vi "MEMR-Export Gain Spectra.vi"(0 "path":path=path "D:/Data/MEMR/Ken/SFMH41-MEMR-1.txt", 7 "processed":T1) -> (15 "error out":errorcluster)   [LabVIEW 2020]
uses:
  Analysis VIs/MEMR-Processed Data.ctl
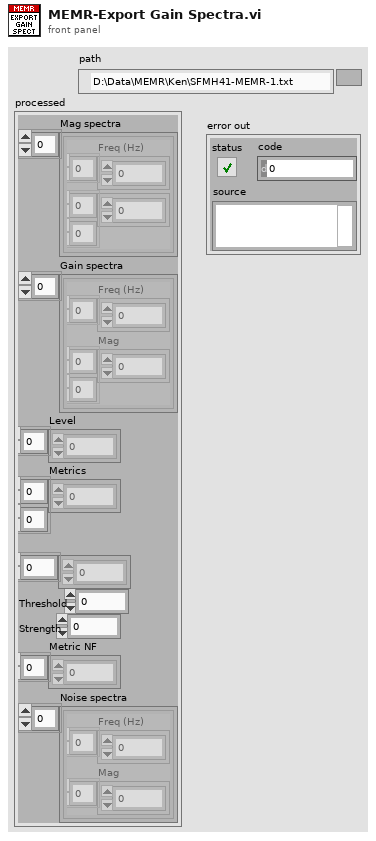
[diagram p1: front panel]
types:
  T1 = typedef "MEMR-Processed Data.ctl" = cluster{"Mag spectra":cluster{"Freq (Hz)":dbl[], dbl[][]}[], "Gain spectra":cluster{"Freq (Hz)":dbl[], "Mag":dbl[][]}[], "Level":dbl[], "Metrics":dbl[][], "Fpeak":dbl[], "Threshold":dbl, "Strength":dbl, "Metric NF":dbl[], "Noise spectra":cluster{"Freq (Hz)":dbl[], "Mag":dbl[]}[]}
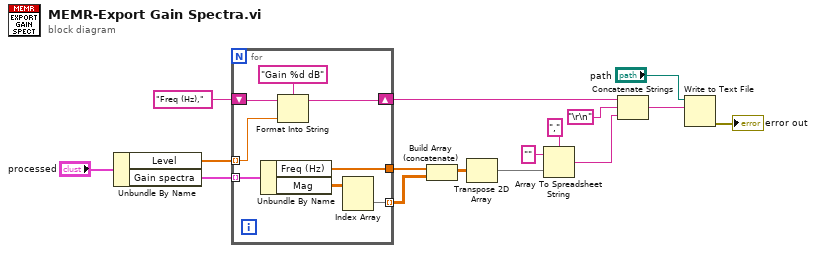
[diagram p0: block diagram]
diagram:
  n1 = Unbundle By Name("processed") -> ("Level"=w14:dbl[], "Gain spectra"=w15:cluster{"Freq (Hz)":dbl[], "Mag":dbl[][]}[])
  n2 = for {
    tunnel: w15 -> [w24] mode=indexing
    tunnel: w14 -> [w19] mode=indexing
    tunnel: [w22] -> w11 mode=indexing
    shift-right: [w20] -> w5
    shift-left: "Freq (Hz)," -> [w21]
    tunnel: [w17] -> w12
    n3 = Unbundle By Name(w24) -> ("Freq (Hz)"=w17:dbl[], "Mag"=w23:dbl[][])
    n4 = Format Into String(format string="Gain %d dB", initial string=w21, w19) -> (resulting string=w20:string)  [unwired: 1 in, 1 out]
    n5 = Index Array(array=w23) -> (element=w22:dbl[])  [unwired: 2 in]
  }
  n6 = Build Array (concatenate)(w12, w11) -> (w10:dbl[][])
  n7 = Transpose 2D Array(2D array=w10) -> (transposed array=w7:dbl[][])
  n8 = Array To Spreadsheet String(delimiter (Tab)=",", array=w7, 3:"" ("format string")) -> (spreadsheet string=w6:string)
  n9 = Concatenate Strings(w5, "\r\n", w6) -> (w3:string)
  n10 = Write to Text File(file (use dialog)="path", text=w3) -> (error out=→"error out":errorcluster)  [unwired: 2 in, 2 out]
